vi "rename_configuration.vi"(8 "error in (no error)":errorcluster, 11 "old name in":string) -> (0 "error out":errorcluster, 2 "canceled?":bool, 3 "new name out":string)   [LabVIEW 2010]
panel:
  in  "button:cancel":bool
  in  "button:done":bool
  in  "new name":string
  out "old name indicator":string caption="old name:"
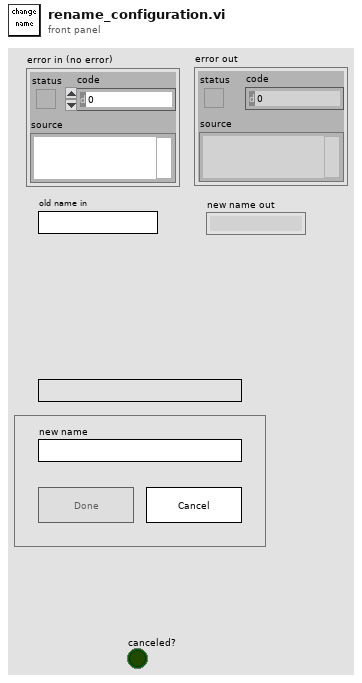
[diagram p1: front panel]
types:
  T1 = enum8{"Enabled", "Disabled", "Disabled and Grayed Out"}
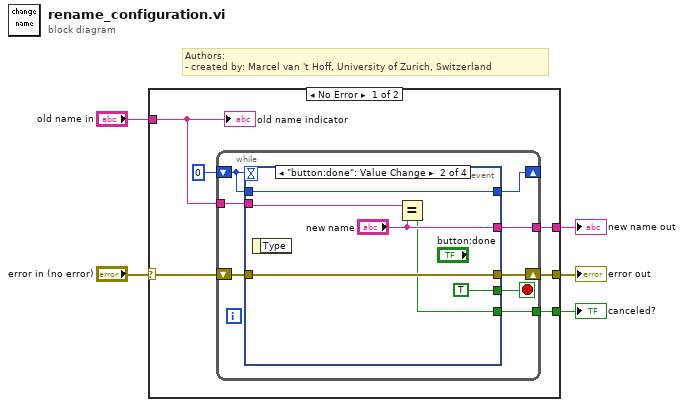
[diagram p0: block diagram]
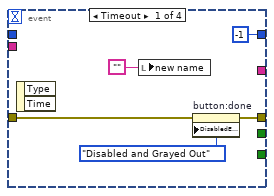
[diagram p2: hidden frame]
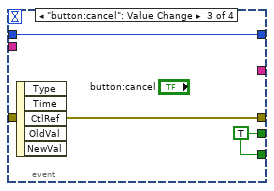
[diagram p3: hidden frame]
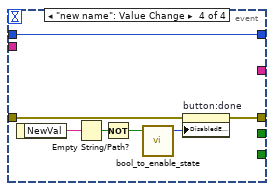
[diagram p4: hidden frame]
diagram:
  # "Authors: \n- created by: Marcel van 't Hoff, University of Zurich, Switzerland"
  n1 = case shown="No Error" "error in (no error)" {
    selector: "error in (no error)" -> [w9 w41]
    tunnel: "old name in" -> [w6 _]
    tunnel: [w11 _] -> w4
    tunnel: [w10 w41] -> w3
    tunnel: [w7 _] -> w1
    frame No Error {
      n2 = while {
        tunnel: [w19] -> w11
        shift-right: [w18] -> w10
        shift-left: w9 -> [w17]
        shift-right: [w14] -> _
        shift-left: 0 -> [w15]
        tunnel: [w13] -> w7
        tunnel: w6 -> [w12]
        stop <- w16 stop-if-true
        n3 = event shown="[1] \"button:done\": Value Change" {
          selector: _ -> [_ _ _ _]
          dyn-events: _ -> [_ _ _ _]
          timeout: w15 -> [_ _ _ _]
          tunnel: [_ "new name" _ _] -> w19
          tunnel: [w22 w30 w33 w38] -> w18
          tunnel: w17 -> [w23 w30 w33 w39]
          tunnel: [_ TRUE w31 _] -> w16
          tunnel: w15 -> [_ w28 w32 w34]
          tunnel: [-1 w28 w32 w34] -> w14
          tunnel: [_ w25 w31 _] -> w13
          tunnel: w12 -> [_ w27 _ _]
          event Timeout {
            n4 = event-data() -> ()  [unwired: 1 in, 2 out]
            n5 = local write "new name"("") -> ()
            n6 = property on="button:done" class="Bool"(error in=w23, "DisabledEnum"=T1."Disabled and Grayed Out" ("Disabled")) -> (error out=w22:errorcluster)  [unwired: 1 in, 1 out]
          }
          event "button:done": Value Change {
            n7 = event-data() -> ()  [unwired: 1 in, 1 out]
            n8 = Equal?(x=w27, y="new name") -> (x = y?=w25:bool)
          }
          event "button:cancel": Value Change {
            w31 = TRUE
            n9 = event-data() -> ()  [unwired: 1 in, 5 out]
          }
          event "new name": Value Change {
            n10 = event-data() -> ("NewVal"=w40:string)  [unwired: 1 in]
            n11 = Empty String/Path?(string/path=w40) -> (empty?=w37:bool)
            n12 = Not(x=w37) -> (.not. x?=w36:bool)
            n13 = call "bool_to_enable_state.vi"("boolean in"=w36) -> ("enabled status out"=w35:T1)  [unwired: 4 in]
            n14 = property on="button:done" class="Bool"(error in=w39, "DisabledEnum"=w35) -> (error out=w38:errorcluster)  [unwired: 1 in, 1 out]
          }
        }
      }
      "old name indicator" <- w6
    }
    frame Error {
    }
  }
  "new name out" <- w4
  "error out" <- w3
  "canceled?" <- w1
